vi "MultipleErrorQuery.vi"(8 "error in (no error)":errorcluster {"code" format="%.0x"}, 11 "instrument handle":refnum<k15>) -> (0 "error out":errorcluster {"code" format="%.0x"}, 2 "Error String":string, 3 "instrument handle out":refnum<k15>)   [LabVIEW 2014]
doc: "Retrieves all error messages."
uses:
  <instrlib>/Agilent NA/Agilent NA.lvlib
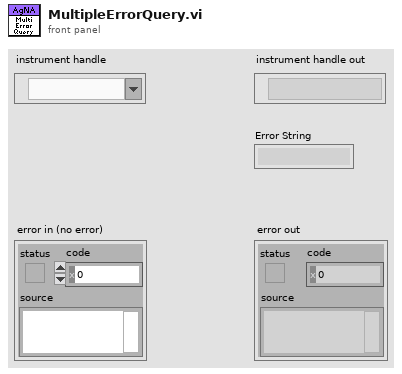
[diagram p1: front panel]
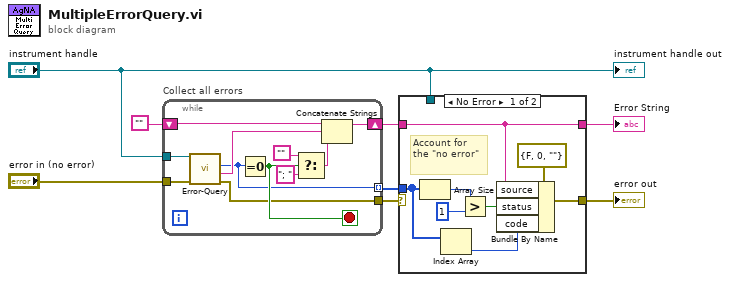
[diagram p0: block diagram]
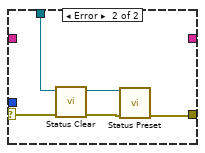
[diagram p2: hidden frame]
diagram:
  n1 = while "Collect all errors" {
    tunnel: "instrument handle" -> [w19]
    shift-right: [w12] -> w5
    shift-left: "" -> [w18]
    tunnel: "error in (no error)" -> [w11]
    tunnel: [w10] -> w4 mode=indexing
    tunnel: [w9] -> w3
    stop <- w16 stop-if-true
    n2 = call <instrlib>:"Error-Query.vi"("error in (no error)"=w11, "instrument handle"=w19) -> ("error out"=w9:errorcluster, "error message"=w17:string, "error code"=w10:i32)  [unwired: 6 in, 1 out]
    n3 = Equal To 0?(x=w10) -> (x = 0?=w16:bool)
    n4 = Select(t="", s=w16, f="; ") -> (s? t:f=w13:string)
    n5 = Concatenate Strings(w18, w17, w13) -> (w12:string)
  }
  n6 = case shown="No Error" w3 {
    selector: w3 -> [_ w32]
    tunnel: [w21 w30] -> w6
    tunnel: w5 -> [w20 _]
    tunnel: w4 -> [w23 _]
    tunnel: [w20 _] -> w2
    tunnel: "instrument handle" -> [_ w29]
    frame No Error {
      # "Account for the \"no error\""
      n7 = Array Size(array=w23) -> (size(s)=w26:i32)
      n8 = Index Array(array=w23) -> (element=w22:i32)  [unwired: 1 in]
      n9 = Greater?(x=w26, y=1) -> (0:w24:bool)
      n10 = Bundle By Name(cluster=errorcluster {"status"=FALSE, "code"=0, "source"=""} ("error out"), "source"=w20, "status"=w24, "code"=w22) -> (w21:errorcluster)
    }
    frame Error {
      n11 = call <instrlib>:"Status Clear.vi"("error in (no error)"=w32, "instrument handle"=w29) -> ("error out"=w31:errorcluster, "instrument handle out"=w28:refnum<k15>)  [unwired: 8 in]
      n12 = call <instrlib>:"Status Preset.vi"("error in (no error)"=w31, "instrument handle"=w28) -> ("error out"=w30:errorcluster)  [unwired: 8 in, 1 out]
    }
  }
  "error out" <- w6
  "Error String" <- w2
  "instrument handle out" <- "instrument handle"
